vi "Global_CMD_ACT_Data In.vi"() -> ()   [LabVIEW 2020, in "Tube Wheel_ACT.lvlib"]
uses:
  roboRIO Code/Systems/Tube Wheel/Tube Wheel_ACT.lvlib
  Cluster_CMD_ACT_Data.ctl
  roboRIO Code/Type Defs/ENUM_TubeWheel_Mode.ctl
  roboRIO Code/Type Defs/ENUM_Tube Wheel CMD Positions.ctl
panel:
  in  "CMD_ACT_TubeWheel_Data":T1 {"Motor speed (0-1)" format="%.3g"}
  # "The Names of the Data items in the Global Variable MUST describe who the Single Writer is\nFor Command Globals the Commander(CMD) represents Teleop or Autonomous or other command loop.\nThe naming convention for a Command Actuator Global is:   \n\nCMD_ACT_SubSystem_Data Name\n\nExample:\nCMD_ACT_Drive_Data\nCMD_ACT_Hopper_Eject Ball"
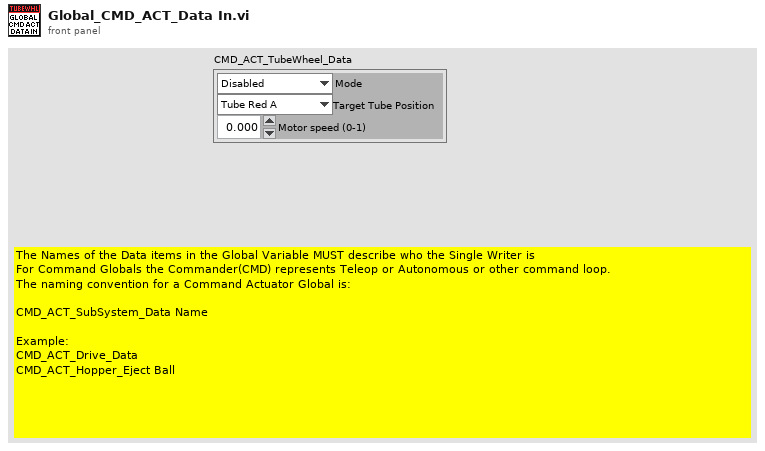
[diagram p1: front panel]
types:
  T1 = typedef "Tube Wheel_ACT.lvlib/Cluster_CMD_ACT_Data.ctl" = cluster{"Mode":T2, "Target Tube Position":T3, "Motor speed (0-1)":dbl}
  T2 = typedef "ENUM_TubeWheel_Mode.ctl" = enum16{"Disabled", "Manual Motor", "Select Positon"}
  T3 = typedef "ENUM_Tube Wheel CMD Positions.ctl" = enum16{"Tube Red A", "Tube Black B", "Tube Red C", "Tube Black D", "Tube Red E", "Tube Black F"}
diagram:
